vi "WPI_DriverStationOutputsEnabled.vi"(8 "error in":errorcluster) -> (0 "error out":errorcluster, 3 "OutputsEnabled?":bool)   [LabVIEW 2017]
doc: "Indicates whether output signals are enabled. Outputs will be disabled due to loss of communications, overvoltage or brownout conditions on the input power to the roboRIO.\n\nThis software is licensed. Open the labview\\readme\\WPI Robotics Library Open Source License.txt file for more information."
uses:
  <vilib>/Utility/error.llb/Error Cluster From Error Code.vi
  <vilib>/rvi/errors/niLvFpgaAdjustHostInterfaceError.vi
  <vilib>/rvi/interface/nirviReadWriteControl/nirviReadWriteControl.xnode
  <vilib>/Rock Robotics/SystemInterfaces/System/FPGA_SystemFRC FPGA Ref.ctl
  NiFpgaLv.dll
  <vilib>/rvi/interface/Simulation/niFpgaSimulationCallBeginRW.vi
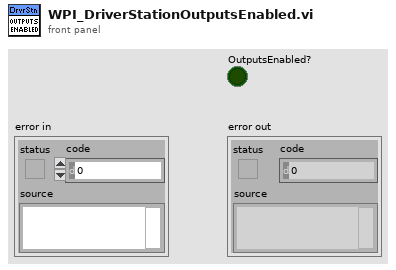
[diagram p1: front panel]
types:
  T1 = typedef "FPGA_SystemFRC FPGA Ref.ctl" = refnum<k20>
  T2 = cluster{"SystemActive":bool, "PowerAlive":bool, "SysDisableCount":fxp<+,15,15>, "PowerDisableCount":fxp<+,15,15>}
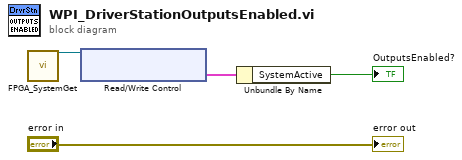
[diagram p0: block diagram]
diagram:
  n1 = call <vilib>:"FPGA_SystemGet.vi"() -> ("FRC FPGA Ref"=w4:T1)  [unwired: 1 in, 10 out]
  n2 = xnode "Read/Write Control"("FPGA VI Reference In"=w4) -> ("SysWatchdog.Status"=w2:T2)  [unwired: 1 in, 2 out]
  n3 = Unbundle By Name(w2) -> ("SystemActive"=→"OutputsEnabled?":bool)
  "error out" <- "error in"
